vi "DoIt.vi"(3 "Rudder":u8(knob)=7, 4 "Prop":u8(slide)=7 scale=0.0..14.0, 5 "IR Servo":u8(knob)=7 scale=0.0..14.0) -> ()   [LabVIEW 2012]
panel:
  out "string":string
  out "error in 2":errorcluster
  out "return count":u32
  out "String Received":string
  out "String":string="$B^"
  in  "error in":errorcluster
  in  "VISA resource name":refnum<visa-resource-name>="COM10"
  out "Heartbeat":bool
  out "Soft Stop\nEngaged":bool
  out "Base\nStation?":bool
  out "Boat?":bool
  in  "SOFT E-STOP":bool
  in  "HARD E-STOP":bool
  in  "# 5":u8 max=5 step=1
  in  "# 4":u8 max=5 step=1
  in  "# 3":u8 max=5 step=1
  in  "# 2":u8 max=5 step=1
  in  "# 1":u8 max=5 step=1
  in  "# 0":u8=1 max=5 step=1
  out "IR Time":dbl
  out "IR Dist":dbl
  # "Behavior\nWeights"
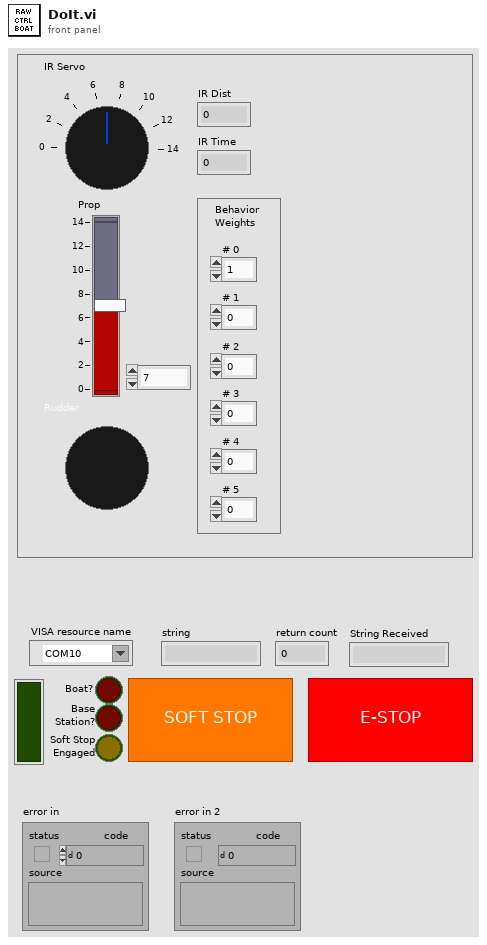
[diagram p1: front panel]
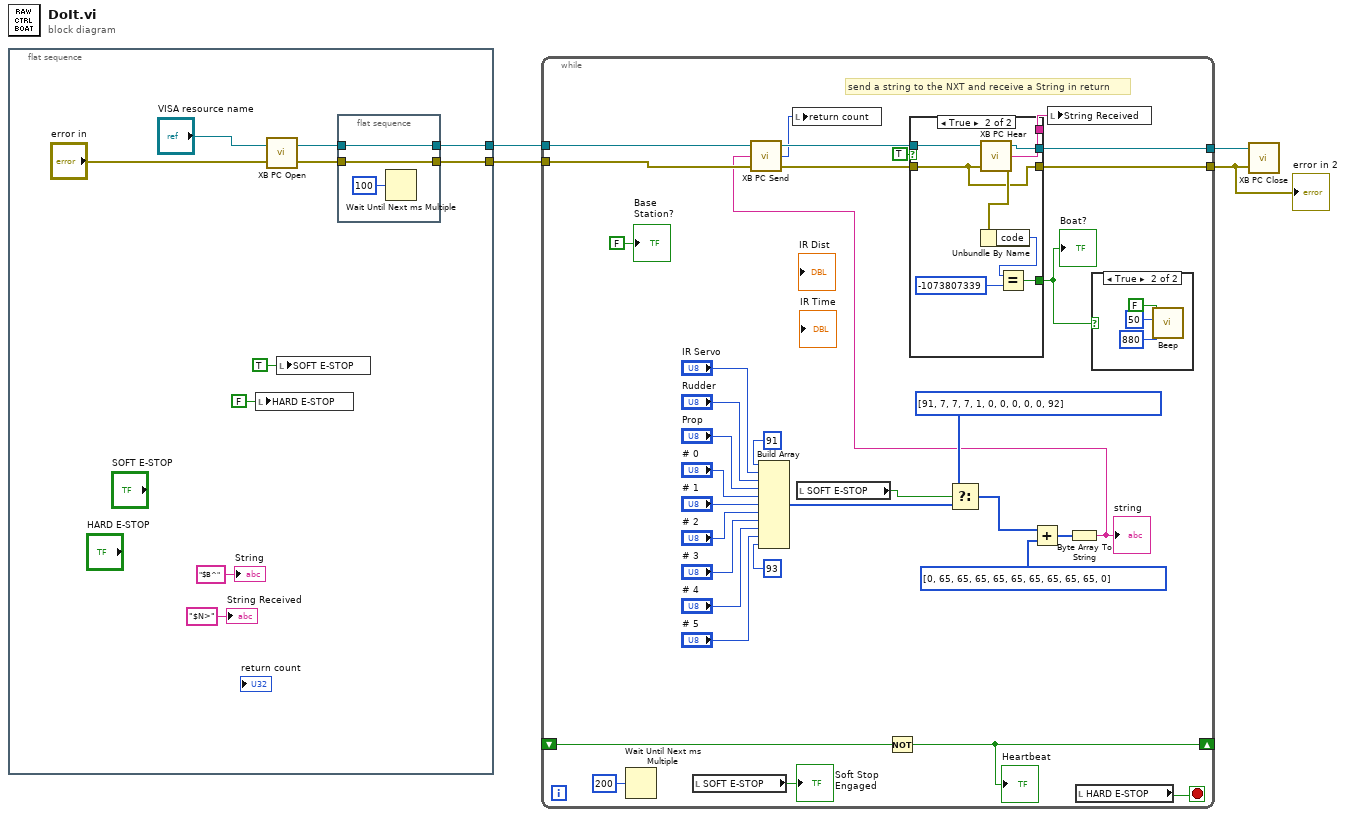
[diagram p0: block diagram]
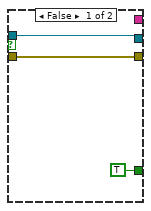
[diagram p3: hidden frame]
diagram:
  n1 = flat-sequence {
    tunnel: [w10] -> w4
    tunnel: [w9] -> w3
    frame #0 {
      n2 = local write "HARD E-STOP"(FALSE ("HARD E-STOP")) -> ()
      n3 = call "XB PC Open.vi"("error in (no error)"="error in", "VISA resource name"="VISA resource name") -> ("error out"=w13:errorcluster, "VISA resource name out"=w14:refnum<visa-resource-name>)
      n4 = local write "SOFT E-STOP"(TRUE ("SOFT E-STOP")) -> ()
      n5 = flat-sequence {
        tunnel: w14 -> [w15]
        tunnel: w13 -> [w16]
        tunnel: [w16] -> w9
        tunnel: [w15] -> w10
        frame #0 {
          n6 = Wait Until Next ms Multiple(millisecond multiple=u32 100) -> ()  [unwired: 1 out]
        }
      }
      "String" <- "$B^" ("String")
      "String Received" <- "$N>" ("String Received")
    }
  }
  n7 = while {
    tunnel: w4 -> [w51]
    tunnel: w3 -> [w50]
    tunnel: [w49] -> w2
    tunnel: [w48] -> w1
    shift-right: [w32] -> _
    shift-left: _ -> [w31]
    stop <- w33 stop-if-true
    # "send a string to the NXT and receive a String in return"
    n8 = Wait Until Next ms Multiple(millisecond multiple=u32 200) -> ()  [unwired: 1 out]
    n9 = local read "SOFT E-STOP"() -> (→"Soft Stop\nEngaged":bool)
    n10 = Build Array(u8 91 ("element"), "IR Servo", "Rudder", "Prop", "# 0", "# 1", "# 2", "# 3", "# 4", "# 5", u8 93 ("element")) -> (w40:u8[])
    n11 = local read "SOFT E-STOP"() -> (w39:bool)
    n12 = Not(x=w31) -> (.not. x?=w32:bool)
    "Heartbeat" <- w32
    n13 = Select(t=u8[] [91, 7, 7, 7, 1, 0, 0, 0, 0, 0, 92], s=w39, f=w40) -> (s? t:f=w28:u8[])
    n14 = Add(x=w28, y=u8[] [0, 65, 65, 65, 65, 65, 65, 65, 65, 65, 0]) -> (x+y=w27:u8[])
    n15 = Byte Array To String(unsigned byte array=w27) -> (string=w21:string)
    "string" <- w21
    n16 = call "XB PC Send.vi"("error in (no error)"=w50, "String"=w21, "VISA resource name"=w51) -> ("error out"=w38:errorcluster, "return count"=w34:u32, "VISA resource name out"=w37:refnum<visa-resource-name>)
    n17 = local write "return count"(w34) -> ()
    n18 = case shown="True" TRUE {
      tunnel: [w57 w65] -> w49
      tunnel: [w56 w58] -> w48
      tunnel: w38 -> [w56 w58]
      tunnel: w37 -> [w57 w64]
      tunnel: [_ w63] -> w35
      tunnel: [TRUE w59] -> w20
      frame False {
      }
      frame True {
        n19 = call "XB PC Hear.vi"("VISA resource name"=w64, "error in (no error)"=w58) -> ("VISA resource name out"=w65:refnum<visa-resource-name>, "String Received"=w63:string, "error out"=w62:errorcluster)
        n20 = Unbundle By Name(w62) -> ("code"=w61:i32)
        n21 = Equal?(x=w61, y=-1073807339) -> (x = y?=w59:bool)
      }
    }
    "Boat?" <- w20
    n22 = local write "String Received"(w35) -> ()
    n23 = local read "HARD E-STOP"() -> (w33:bool)
    n24 = case shown="True" w20 {
      frame False {
      }
      frame True {
        n25 = call <vilib>:"Beep.vi"("use system alert? (T)"=FALSE, "duration (msec)"=u32 50, "frequency (Hz)"=u32 880) -> ()  [unwired: 9 in]
      }
    }
    "Base\nStation?" <- FALSE ("Base\nStation?")
  }
  "error in 2" <- w1
  n26 = call "XB PC Close.vi"("error in (no error)"=w1, "VISA resource name"=w2) -> ()
